vi "Update path.vi"(1 "Support Directory Name (EXE)":string="Data", 3 "Path IN":path) -> (0 "Path OUT":path)   [LabVIEW 2020, in "Exaprom PDF.lvlib"]
doc: "Update the path for different versions of LV."
uses:
  <userlib>/labview-PDF-writer-master/Exaprom PDF.lvlib
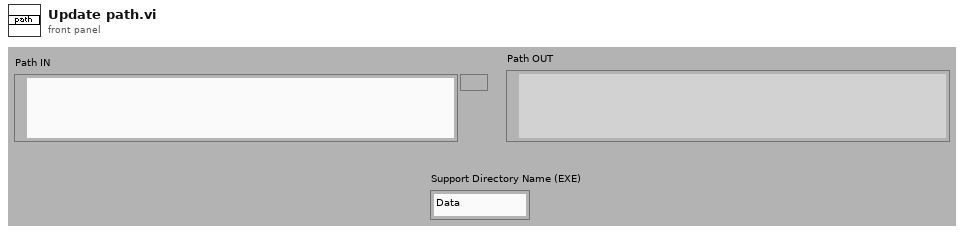
[diagram p1: front panel]
types:
  T1 = enum32{"invalid app kind", "Development System", "Run Time System", "Student Edition", "Embedded LabVIEW", "Evaluation", "Custom"}
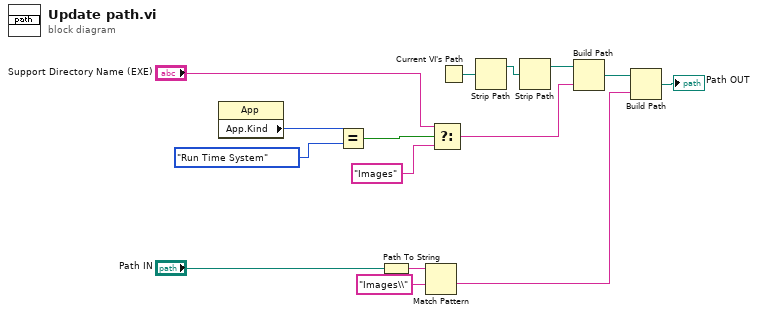
[diagram p0: block diagram]
diagram:
  n1 = property class="App"() -> ("App.Kind"=w10:T1)  [unwired: 2 in, 2 out]
  n2 = Equal?(x=w10, y=T1."Run Time System") -> (x = y?=w7:bool)
  n3 = Path To String(path="Path IN") -> (string=w3:string)
  n4 = Match Pattern(string=w3, regular expression="Images\\") -> (after substring=w1:string)  [unwired: 1 in, 3 out]
  n5 = Select(t="Support Directory Name (EXE)", s=w7, f="Images" ("name or relative path")) -> (s? t:f=w5:string)
  n6 = Current VI's Path() -> (path=w15:path)
  n7 = Strip Path(path=w15) -> (stripped path=w14:path)  [unwired: 1 out]
  n8 = Strip Path(path=w14) -> (stripped path=w13:path)  [unwired: 1 out]
  n9 = Build Path(base path=w13, name or relative path=w5) -> (appended path=w12:path)
  n10 = Build Path(base path=w12, name or relative path=w1) -> (appended path=→"Path OUT":path)
